vi "doPygmentization on VI.vi"(0 "Text Field Destination":refnum<vi>, 1 "style name (material)":string="material", 2 "Type":string, 7 "String":string) -> ()   [LabVIEW 2026]
uses:
  Text Style Definition.ctl
  <vilib>/regexp/Match Regular Expression.xnode
panel:
  out "error out":errorcluster
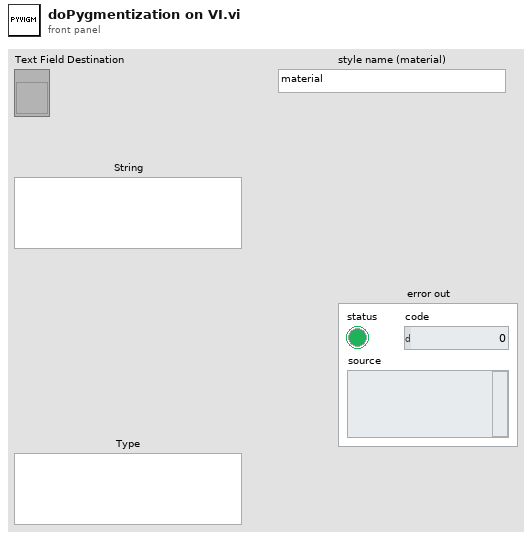
[diagram p1: front panel]
types:
  T1 = cluster{"Python version":string[], "Python version":string[]}
  T2 = typedef "Text Style Definition.ctl" = cluster{"FG color":u32, "bold":bool, "italic":bool, "underline":bool, "roman":bool, "sans":bool, "mono":bool, "strikethrough":bool, "BG color":u32}
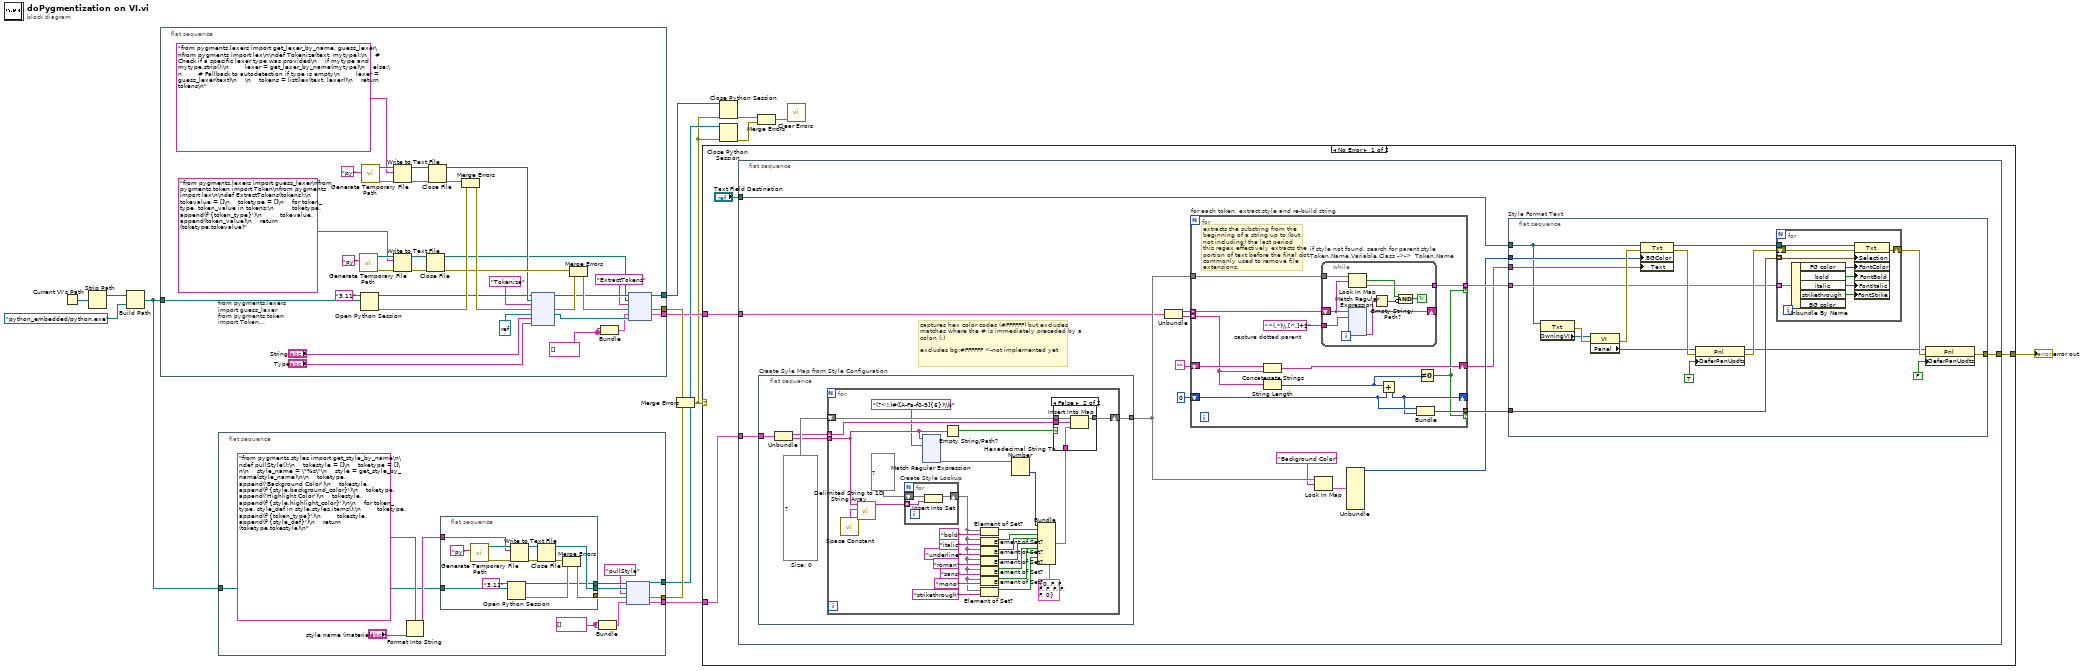
[diagram p0: block diagram]
diagram:
  n1 = Current VI's Path() -> (path=w4:path)
  n2 = Strip Path(path=w4) -> (stripped path=w2:path)  [unwired: 1 out]
  n3 = Build Path(base path=w2, name or relative path=path "python_embedded/python.exe" ("python path")) -> (appended path=w1:path)
  n4 = flat-sequence {
    tunnel: [w42] -> w12
    tunnel: [w23] -> w14
    tunnel: w1 -> [w19]
    tunnel: [w18] -> w10
    frame #0 {
      w20 = "from pygments.lexers import guess_lexer\nfrom pygments.token import Token\nfrom pygments import lex\n\ndef ExtractTokens(tokens):\n    tokevalue = []\n    toketype = []\n    for token_type, token_value in tokens:\n         toketype.append(f'{token_type}')\n         tokevalue.append(token_value)\n    return (toketype,tokevalue)"  # from pygments.lexers import guess_lexer from pygments.token import Token from pygments import lex  def ExtractTokens(tokens):     tokevalue = []     toketype = []     for token_type, token_value in tokens:          toketype.append(f'{token_type}')          tokevalue.append(token_value)     return (toketype,tokevalue)
      w21 = string[] [] ("Python version")
      n5 = call <vilib>:"Generate Temporary File Path.vi"("Temporary File Extension (tmp)"="py") -> ("error out"=w47:errorcluster, "Unique Temporary File Path"=w35:path)  [unwired: 9 in]
      n6 = Open Python Session(python version="3.11" ("Python version"), python path=w19) -> (session out=w30:refnum<k35>, error out=w45:errorcluster)  [unwired: 1 in]
      n7 = call <vilib>:"Generate Temporary File Path.vi"("Temporary File Extension (tmp)"="py") -> ("error out"=w48:errorcluster, "Unique Temporary File Path"=w36:path)  [unwired: 9 in]
      n8 = Write to Text File(file (use dialog)=w36, text="from pygments.lexers import get_lexer_by_name, guess_lexer\nfrom pygments import lex\n\ndef Tokenize(text, mytype):\n    # Check if a specific lexer type was provided\n    if mytype and mytype.strip():\n        lexer = get_lexer_by_name(mytype)\n    else:\n        # Fallback to autodetection if type is empty\n        lexer = guess_lexer(text)\n    \n    tokens = list(lex(text, lexer))\n    return tokens\n", error in=w48) -> (refnum out=w39:refnum<file>, error out=w49:errorcluster)  [unwired: 1 in, 1 out]
      n9 = Write to Text File(file (use dialog)=w35, text=w20, error in=w47) -> (refnum out=w33:refnum<file>, error out=w46:errorcluster)  [unwired: 1 in, 1 out]
      n10 = Close File(refnum=w33, error in=w46) -> (path=w27:path, error out=w43:errorcluster)
      n11 = Close File(refnum=w39, error in=w49) -> (path=w31:path, error out=w50:errorcluster)
      n12 = Merge Errors(w50, w45) -> (w44:errorcluster)
      n13 = node(w30, w31, "Tokenize" ("function name"), w44, refnum<k38> refnum ("Python Object Refnum"), "String", "Type") -> (w32:refnum<k35>, w41:errorcluster, w25:refnum<k38>)  [unwired: 2 in, 2 out]
      n14 = Merge Errors(w43, w41) -> (w40:errorcluster)
      n15 = Bundle("Python version"=w21, "Python version"=w21) -> (w22:T1)  [unwired: 1 in]
      n16 = node(w32, w27, "ExtractTokens" ("function name"), w40, w22, w25) -> (w18:refnum<k35>, w42:errorcluster, w23:T1)  [unwired: 1 in, 2 out]
    }
  }
  n17 = flat-sequence {
    tunnel: [w58] -> w15
    tunnel: [w53] -> w11
    tunnel: w1 -> [w52]
    tunnel: [w51] -> w9
    frame #0 {
      w57 = string[] [] ("Python version")
      n18 = Format Into String(format string="from pygments.styles import get_style_by_name\n\ndef pullStyle():\n    tokestyle = []\n    toketype = []\n\n    style_name = \"%s\"\n    style = get_style_by_name(style_name)\n\n    toketype.append('Background Color')\n    tokestyle.append(f'{style.background_color}')\n    toketype.append('Highlight Color')\n    tokestyle.append(f'{style.highlight_color}')\n\n    for token_type, style_def in style.styles.items():\n        toketype.append(f'{token_type}')\n        tokestyle.append(f'{style_def}')\n    return (toketype,tokestyle)\n" ("text"), "style name (material)") -> (resulting string=w55:string)  [unwired: 2 in, 1 out]
      n19 = flat-sequence {
        tunnel: [w67] -> w62
        tunnel: [w66] -> w61
        tunnel: [w72] -> w63
        tunnel: w55 -> [w65]
        tunnel: w52 -> [w64]
        frame #0 {
          n20 = call <vilib>:"Generate Temporary File Path.vi"("Temporary File Extension (tmp)"="py") -> ("error out"=w76:errorcluster, "Unique Temporary File Path"=w69:path)  [unwired: 9 in]
          n21 = Open Python Session(python version="3.11" ("Python version"), python path=w64) -> (session out=w66:refnum<k35>, error out=w73:errorcluster)  [unwired: 1 in]
          n22 = Write to Text File(file (use dialog)=w69, text=w65, error in=w76) -> (refnum out=w68:refnum<file>, error out=w75:errorcluster)  [unwired: 1 in, 1 out]
          n23 = Close File(refnum=w68, error in=w75) -> (path=w67:path, error out=w74:errorcluster)
          n24 = Merge Errors(w74, w73) -> (w72:errorcluster)
        }
      }
      n25 = Bundle("Python version"=w57, "Python version"=w57) -> (w59:T1)  [unwired: 1 in]
      n26 = node(w61, w62, "pullStyle" ("function name"), w63, w59) -> (w51:refnum<k35>, w53:errorcluster, w58:T1)  [unwired: 2 out]
    }
  }
  n27 = Merge Errors(w12, w11) -> (w8:errorcluster)
  n28 = case shown="No Error" w8 {
    selector: w8 -> [_ w421]
    tunnel: w15 -> [w80 _]
    tunnel: w14 -> [w79 _]
    tunnel: [w77 w421] -> w13
    frame No Error {
      n29 = flat-sequence {
        tunnel: w80 -> [w92]
        tunnel: w79 -> [w87]
        tunnel: "Text Field Destination" -> [w85]
        tunnel: [w82] -> w77
        frame #0 {
          # "captures hex color codes (#FFFFFF) but excludes matches where the # is immediately preceded by a colon (:)\n\nexcludes bg:#FFFFFF <-not implemented yet"
          n30 = flat-sequence "Create Syle Map from Style Configuration" {
            tunnel: [w126] -> w90
            tunnel: w92 -> [w124]
            frame #0 {
              w125 = map{string, T2} {}  # Size: 0
              n31 = Unbundle(w124) -> ("Python version"=w123:string[], "Python version"=w122:string[])
              n32 = for {
                tunnel: w123 -> [w135] mode=indexing
                shift-right: [w154] -> w126
                shift-left: w125 -> [w153]
                tunnel: w122 -> [w132] mode=indexing
                n33 = call <vilib>:"Space Constant.vi"() -> ("String"=w152:string)
                n34 = call <vilib>:"Delimited String to 1D String Array.vi"("delimiter"=w152, "delimited string"=w132) -> ("string array"=w133:string[])  [unwired: 9 in]
                n35 = for "Create Style Lookup" {
                  tunnel: w133 -> [w280] mode=indexing
                  shift-right: [w279] -> w128
                  shift-left: set{string} {} ("set") -> [w281]
                  n36 = Insert Into Set(10:w280, 11:w281) -> (3:w279:set{string})  [unwired: 1 out]
                }
                n37 = xnode "Match Regular Expression"("input string"=w132, "regular expression"="(?<!:)#([A-Fa-f0-9]{6})\\b") -> ("submatch 1"=w130:string)  [unwired: 4 in, 5 out]
                n38 = Empty String/Path?(string/path=w132) -> (empty?=w134:bool)
                n39 = Element of Set?(10:"bold", 11:w128) -> (3:w144:bool)
                n40 = Element of Set?(10:"italic", 11:w128) -> (3:w143:bool)
                n41 = Element of Set?(10:"underline", 11:w128) -> (3:w142:bool)
                n42 = Element of Set?(10:"roman", 11:w128) -> (3:w138:bool)
                n43 = Element of Set?(10:"sans", 11:w128) -> (3:w141:bool)
                n44 = Element of Set?(10:"mono", 11:w128) -> (3:w140:bool)
                n45 = Element of Set?(10:"strikethrough", 11:w128) -> (3:w127:bool)
                n46 = Hexadecimal String To Number(string=w130) -> (number=w151:u32)  [unwired: 2 in, 1 out]
                n47 = Bundle(cluster=T2 {"FG color"=0, "bold"=FALSE, "italic"=FALSE, "underline"=FALSE, "roman"=FALSE, "sans"=FALSE, "mono"=FALSE, "strikethrough"=FALSE, "BG color"=0}, "FG color"=w151, "bold"=w144, "italic"=w143, "underline"=w142, "roman"=w138, "sans"=w141, "mono"=w140, "strikethrough"=w127) -> (w139:T2)  [unwired: 1 in]
                n48 = case shown="False" w134 {
                  tunnel: w135 -> [_ w278]
                  tunnel: [w274 w277] -> w154
                  tunnel: w153 -> [w274 w276]
                  tunnel: w139 -> [_ w275]
                  frame True {
                  }
                  frame False {
                    n49 = Insert Into Map(map in=w276, key=w278, value=w275) -> (map out=w277:map{string, T2})  [unwired: 2 out]
                  }
                }
              }
            }
          }
          n50 = Unbundle(w87) -> ("Python version"=w84:string[], "Python version"=w83:string[])
          n51 = for "for each token, extract style and re-build string" {
            tunnel: w90 -> [w293]
            shift-right: [w287] -> _
            shift-left: 0 ("length") -> [w288]
            shift-right: [w286] -> w86
            shift-left: "" ("function name 2") -> [w292]
            tunnel: [w290] -> w93 mode=indexing if=w282
            tunnel: [w291] -> w95 mode=indexing if=w282
            tunnel: w84 -> [w285] mode=indexing
            tunnel: w83 -> [w284] mode=indexing
            w289 = "^(.*)\\.[^.]+$"  # capture dotted parent
            # "extracts the substring from the beginning of a string up to (but not including) the last period\nthis regex effectively extracts the portion of text before the final dot, commonly used to remove file extensions."
            n52 = Concatenate Strings(w292, w284) -> (w286:string)
            n53 = String Length(string=w284) -> (length=w283:i32)
            n54 = while "if style not found, search for parent style\nToken.Name.Variable.Class ->->  Token.Name" {
              tunnel: w293 -> [w301]
              tunnel: [w300] -> w291
              shift-right: [w294] -> _
              shift-left: w285 -> [w299]
              tunnel: w289 -> [w297]
              stop <- w298 continue-if-true
              n55 = Look In Map(map=w301, key=w299) -> (key not found?=w295:bool, value=w300:T2)  [unwired: 1 in]
              n56 = xnode "Match Regular Expression"("input string"=w299, "regular expression"=w297) -> ("submatch 1"=w294:string)  [unwired: 4 in, 5 out]
              n57 = Empty String/Path?(string/path=w294) -> (empty?=w296:bool)
              n58 = Compound Arithmetic op=AND(w295, invert w296) -> (w298:bool)
            }
            n59 = Add(x=w283, y=w288) -> (x+y=w287:i32)
            n60 = Bundle("length"=w288, w287) -> (w290:cluster{"length":i32, i32})  [unwired: 1 in]
            n61 = Not Equal To 0?(x=w283) -> (x != 0?=w282:bool)
          }
          n62 = Look In Map(map=w90, key="Background Color") -> (value=w91:T2)  [unwired: 1 in, 1 out]
          n63 = Unbundle(w91) -> ("FG color"=w88:u32)  [unwired: 8 out]
          n64 = flat-sequence "Style Format Text" {
            tunnel: w93 -> [w107]
            tunnel: w88 -> [w106]
            tunnel: w86 -> [w97]
            tunnel: w95 -> [w102]
            tunnel: w85 -> [w98]
            tunnel: [w96] -> w82
            frame #0 {
              n65 = property class="Txt"(reference=w98) -> (error out=w108:errorcluster, "OwningVI"=w101:refnum<vi>)  [unwired: 1 in, 1 out]
              n66 = property class="VI"(reference=w101, error in=w108) -> (error out=w110:errorcluster, "Panel"=w104:refnum<vi>)  [unwired: 1 out]
              n67 = property class="Txt"(reference=w98, error in=w110, "BGColor"=w106, "Text"=w97) -> (reference out=w103:refnum<vi>, error out=w109:errorcluster)
              n68 = property class="Pnl"(reference=w104, error in=w109, "DeferPanUpdts"=TRUE ("Defer Panel Updates")) -> (reference out=w105:refnum<vi>, error out=w112:errorcluster)
              n69 = for {
                tunnel: w103 -> [w120]
                tunnel: w107 -> [w119] mode=indexing
                tunnel: w102 -> [w118] mode=indexing
                shift-right: [w121] -> w111
                shift-left: w112 -> [w115]
                n70 = Unbundle By Name(w118) -> ("FG color"=w117:u32, "bold"=w114:bool, "italic"=w113:bool, "strikethrough"=w116:bool)  [unwired: 1 out]
                n71 = property class="Txt"(reference=w120, error in=w115, "Selection"=w119, "FontColor"=w117, "FontBold"=w114, "FontItalic"=w113, "FontStrike"=w116) -> (error out=w121:errorcluster)  [unwired: 1 out]
              }
              n72 = property class="Pnl"(reference=w105, error in=w111, "DeferPanUpdts"=FALSE ("Defer Panel Updates")) -> (error out=w96:errorcluster)  [unwired: 1 out]
            }
          }
        }
      }
    }
    frame Error {
    }
  }
  "error out" <- w13
  n73 = Close Python Session(session in=w10, error in=w8) -> (11:w7:errorcluster)
  n74 = Close Python Session(session in=w9, error in=w8) -> (11:w6:errorcluster)
  n75 = Merge Errors(w7, w6) -> (w5:errorcluster)
  n76 = call <vilib>:"Clear Errors.vi"("error in (no error)"=w5) -> ()  [unwired: 5 in, 2 out]
